vi "Read LS 331.vi"() -> ()   [LabVIEW 2017]
uses:
  <instrlib>/Lake Shore Cryotronics 331/Lake Shore Cryotronics 331.lvlib
panel:
  in  "ID Query (True)":bool
  in  "?":u16(ring) items=["Kelvin", "Celsius", "Sensor Units"]
  in  "Sensor Input (0:A)":u16(ring) items=["A", "B"]
  out "error out":errorcluster
  in  "error in (no error)":errorcluster
  out "Sensor Data":dbl format="%.4f"
  in  "Serial Configuration":T1={"Baud Rate"=9600, "Parity"=1, "Data Bits"=7, "Stop Bits"=10, "Flow Control"=0} {"Flow Control" items=["None", "XON/XOFF", "RTS/CTS", "XON/XOFF & RTS/CTS", "DTR/DSR", "XON/XOFF & DTR/DSR"]; "Stop Bits" items=["1.0"=10, "1.5"=15, "2.0"=20]; "Data Bits" items=["7"=7, "8"=8]; "Parity" items=["None", "Odd", "Even", "Mark", "Space"]; "Baud Rate" items=["300"=300, "600"=600, "1200"=1200, "2400"=2400, "4800"=4800, "9600"=9600, "19200"=19200, "38400"=38400, "57600"=57600]}
  in  "325 VISA resource":refnum<visa-resource-name>="COM22"
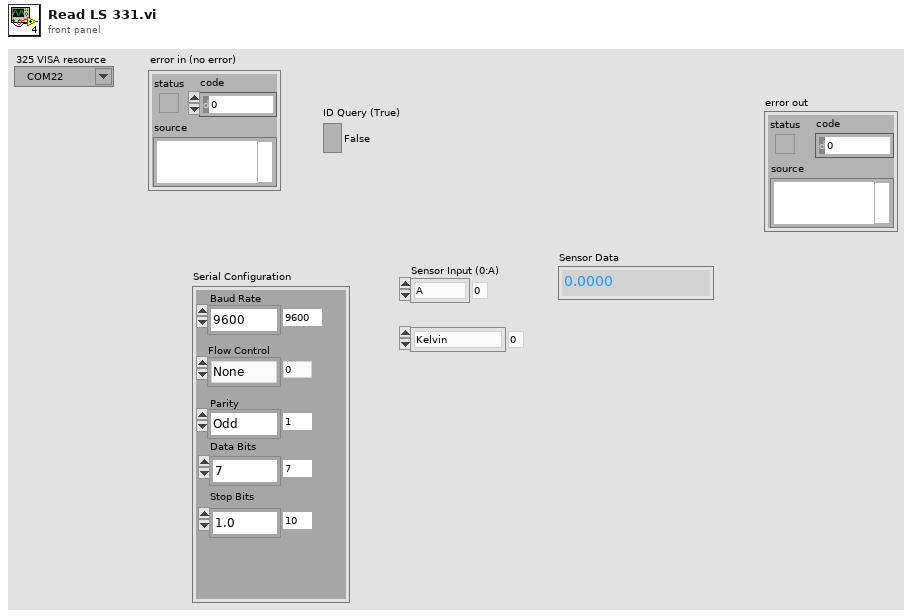
[diagram p1: front panel]
types:
  T1 = cluster{"Baud Rate":u32, "Parity":u16, "Data Bits":u16, "Stop Bits":u16, "Flow Control":u16}
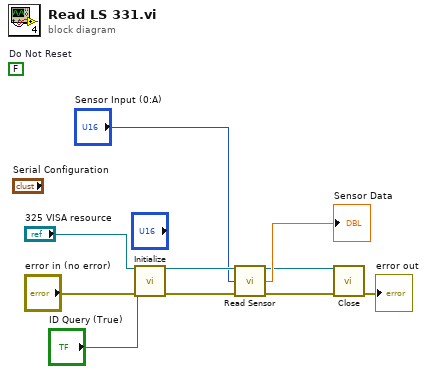
[diagram p0: block diagram]
diagram:
  (unwired) FALSE  # Do Not Reset
  n1 = call <instrlib>:"Initialize.vi"("VISA resource name"="325 VISA resource", "ID Query (True)"="ID Query (True)", "error in (no error)"="error in (no error)") -> ("VISA resource name out"=w6:refnum<visa-resource-name>, "error out"=w7:errorcluster)  [unwired: 11 in]
  n2 = call <instrlib>:"Read Sensor.vi"("VISA resource name"=w6, "Input (0: A)"="Sensor Input (0:A)", "error in (no error)"=w7) -> ("VISA resource name out"=w4:refnum<visa-resource-name>, "Kelvin Reading"=→"Sensor Data":dbl, "error out"=w3:errorcluster)  [unwired: 8 in, 2 out]
  n3 = call <instrlib>:"Close.vi"("VISA resource name"=w4, "error in (no error)"=w3) -> ("error out"=→"error out":errorcluster)  [unwired: 13 in]
